vi "Save Channel response to CSV.vi"(8 "error in (no error)":T2, 10 "channel":T1, 11 "Path":path) -> (0 "error out":T2)   [LabVIEW 2019]
uses:
  <vilib>/Utility/file.llb/Write Delimited Spreadsheet (string).vi
  <vilib>/Utility/file.llb/Write Delimited Spreadsheet (DBL).vi
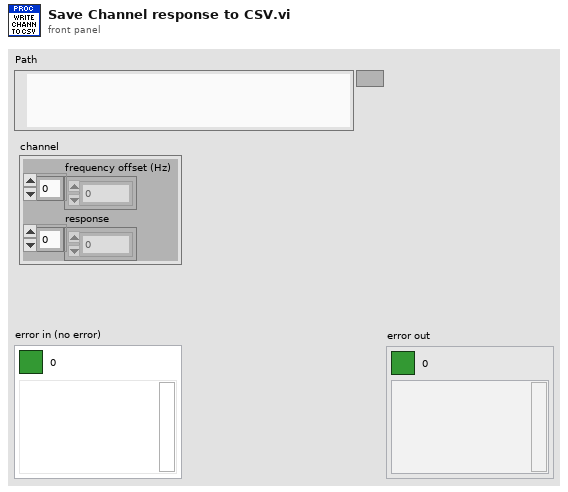
[diagram p1: front panel]
types:
  T1 = cluster{"frequency offset (Hz)":dbl[], "response":cdb[]}
  T2 = cluster{"Boolean Round":bool, "code":i32, "source":string}
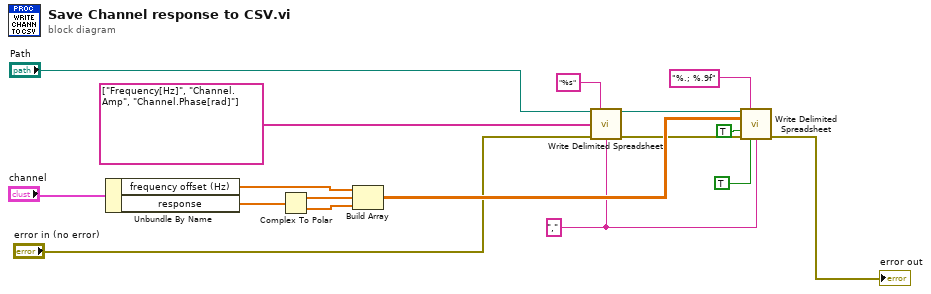
[diagram p0: block diagram]
diagram:
  w4 = "," ("delimiter (\\t)")
  n1 = Unbundle By Name("channel") -> ("frequency offset (Hz)"=w1:dbl[], "response"=w2:cdb[])
  n2 = Complex To Polar(r * e^(i*theta)=w2) -> (r=w17:dbl[], theta=w16:dbl[])
  n3 = Build Array(w1, w17, w16) -> (w10:dbl[][])
  n4 = call-poly <vilib>:"Write Delimited Spreadsheet.vi"("file path (dialog if empty)"="Path", "format (%s)"="%s" ("format (%.3f)"), "1D data"=string[] ["Frequency[Hz]", "Channel.Amp", "Channel.Phase[rad]"] ("format (%.3f)"), "error in (no error)"="error in (no error)", "delimiter (\\t)"=w4) -> ("new file path (Not A Path if cancelled)"=w11:path, "error out"=w6:errorcluster)  [unwired: 9 in]
  n5 = call-poly <vilib>:"Write Delimited Spreadsheet.vi"("file path (dialog if empty)"=w11, "format (%.3f)"="%.; %.9f" ("format string"), "2D data"=w10, "append to file? (new file:F)"=TRUE, "error in (no error)"=w6, "transpose? (no:F)"=TRUE, "delimiter (\\t)"=w4) -> ("error out"=→"error out":errorcluster)  [unwired: 7 in, 1 out]
